vi "Insert Stop Message.vi"(8 "error in (no error)":errorcluster, 11 "BehaviorData in":refnum<class "BehaviorData.lvclass">) -> (0 "error out":errorcluster, 3 "BehaviorData out":refnum<class "BehaviorData.lvclass">)   [LabVIEW 2014, in "BehaviorData.lvclass"]
uses:
  BehaviorData.lvclass
  Database/BehPrimary.ctl
  AcquistionObject/AcquistionObject.lvclass
panel:
  out "resulting string":string
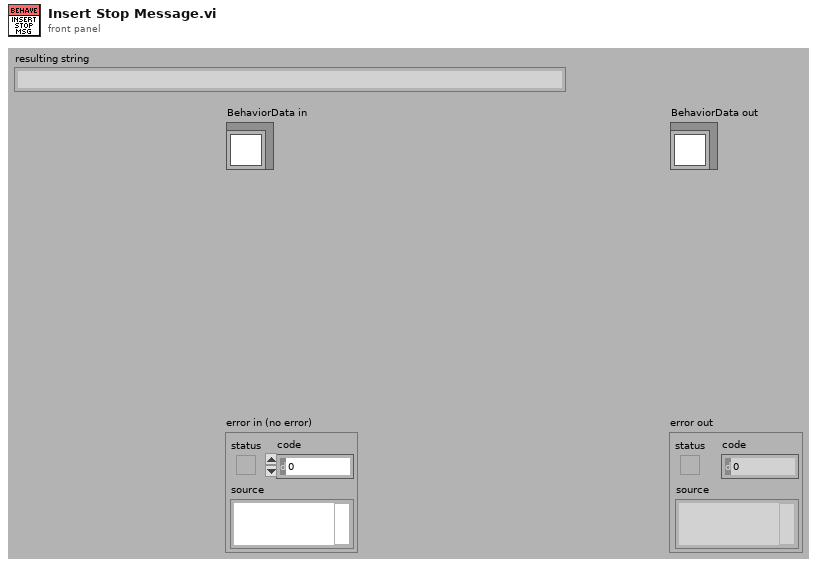
[diagram p1: front panel]
types:
  T1 = typedef "BehPrimary.ctl" = cluster{"setup":u8, "subject_id":i32, "session_start_time":dbl, "stim_start_time":dbl}
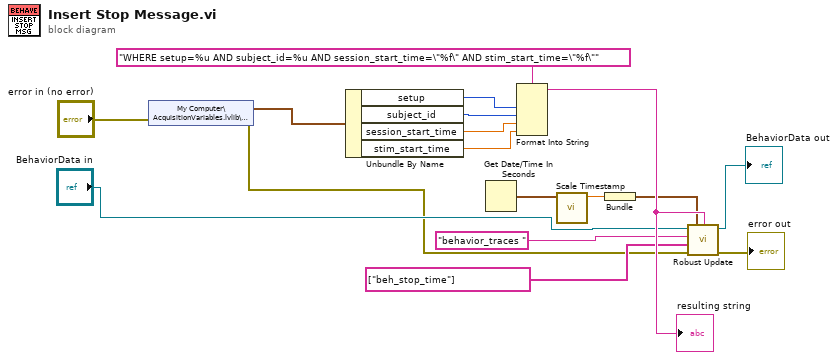
[diagram p0: block diagram]
diagram:
  n1 = shared-variable "My Computer\\AcquisitionVariables.lvlib\\BehaviorPK"(error in="error in (no error)") -> (w16:T1, error out=w2:errorcluster)
  n2 = Unbundle By Name(w16) -> ("setup"=w14:u8, "subject_id"=w13:i32, "session_start_time"=w11:dbl, "stim_start_time"=w9:dbl)
  n3 = Get Date/Time In Seconds() -> (seconds since 1Jan1904=w17:timestamp)
  n4 = Format Into String(format string="WHERE setup=%u AND subject_id=%u AND session_start_time=\"%f\" AND stim_start_time=\"%f\"", w14, w13, w11, w9) -> (resulting string=w7:string)  [unwired: 2 in, 1 out]
  "resulting string" <- w7
  n5 = call "Scale Timestamp.vi"("Time Stamp"=w17) -> ("Scaled timestamp"=w12:dbl)  [unwired: 10 in]
  n6 = Bundle("Scaled timestamp"=w12) -> (w6:cluster{"Scaled timestamp":dbl})  [unwired: 1 in]
  n7 = call "Robust Update.vi"("condition"=w7, "data"=w6, "error in (no error)"=w2, "columns"=string[] ["beh_stop_time"], "table"="behavior_traces ", "AcquistionObject.lvclass"="BehaviorData in") -> ("error out"=→"error out":errorcluster, "AcquistionObject out"=→"BehaviorData out":refnum<class "BehaviorData.lvclass">)  [unwired: 4 in]
